vi "WriteFlashFile 3.vi"(0 "Input File Path":path=path "C:/Program Files/WinLapss/Data/4-7-10 2J Anneal Tests/B-615-4-A780_tbilir_Flash-9-5768.dat", 1 "IV array":dbl[][](array[numeric])=[[-0.00396842, -0.00400707, -0.00401566, -0.00399848, -0.00400707, -0.00402855, -0.00398989, -0.00399848, -0.00403713, -0.00402424, -0.00400277, -0.00401137, -0.00396842, -0.00401137, -0.00401566, -0.00395553, -0.00401995, -0.00401995, -0.00400277, -0.00401566, -0.0039856, -0.00401566, -0.00395983, -0.00403284, -0.00400707, -0.00401137, -0.00401137, -0.0039856, -0.00395553, -0.00399419, -0.00403713, -0.00402855, -0.00401995, -0.00397271, -0.0040586, -0.00403713, -0.00396842, -0.00400277, -0.0039813, -0.00404572, -0.0039813, -0.0039856, -0.00403713, -0.00405002, -0.00399848, -0.00399419, -0.00407149, -0.0039813, -0.00402855, -0.00402855, -0.00397701, -0.00399419, -0.00404142, -0.00400707, -0.00399419, -0.00399848, -0.00398989, -0.00400277, -0.00401995, -0.00398989, -0.00402855, -0.00404142, -0.00403713, -0.00404572, -0.00404572, -0.00397271, -0.00399848, -0.00402424, -0.00398989, -0.00403713, -0.00404142, -0.0039813, -0.00402424, -0.00400277, -0.0039813, -0.00402855, -0.00402424, -0.00400277, -0.00404572, -0.00398989, -0.00401137, -0.00400707, -0.00403284, -0.00401995, -0.00408866, -0.00398989, -0.00395553, -0.00395553, -0.00395983, -0.0039856, -0.0039856, -0.00402424, -0.00402855, -0.00401995, -0.00402855, -0.00401995, -0.00402855, -0.00392117, -0.00394266, -0.00399848, -0.00397271, -0.00396413, -0.00403713, -0.00397271, -0.00401137, -0.00404572, -0.00400707, -0.00395553, -0.00401137, -0.00393406, -0.00397701, -0.00405431, -0.0039856, -0.00394266, -0.00402424, -0.00399848, -0.00400707, -0.00403713, -0.00401995, -0.00398989, -0.00400707, -0.00398989, -0.00399848, -0.00397271, -0.00397271, -0.00401137, -0.00402855, -0.00398989, -0.0039813, -0.00399848, -0.00402855, -0.00400707, -0.00407149, -0.00405002, -0.00403284, -0.00401566, -0.00401566, -0.00400277, -0.00401137, -0.00398989, -0.00394695, -0.0039813, -0.00392977, -0.0039856, -0.00398989, -0.00397271, -0.00400277, -0.0039856, -0.00401566, -0.00400707, -0.0039856, -0.00392117, -0.00400277, -0.00398989, -0.00397271, -0.00396413, -0.00397701, -0.00399848, -0.00400277, -0.00395124, -0.00395983, -0.00396413, -0.00396842, -0.00402424, -0.00398989, -0.0039813, -0.00399848, -0.00399848, -0.00394266, -0.00394695, -0.00400707, -0.00401995, -0.00404142, -0.00396413, -0.00400277, -0.00393835, -0.00402855, -0.0039856, -0.0039856, -0.00404572, -0.00400277, -0.00397701, -0.00397701, -0.00396842, -0.00401566, -0.00397271, -0.0039856, -0.00401566, -0.00395124, -0.00400277, -0.00401995, -0.00399419, -0.0039813, -0.00400277, -0.00399848, -0.00396842, -0.00397271, -0.00397271, -0.00396842, -0.00399419, -0.00392117, -0.00392977, -0.0039856, -0.00394266, -0.00395553, -0.00400277, -0.00393406, -0.00396413, -0.00395553, -0.00387824, -0.00393835, -0.00397701, -0.00392548, -0.00395124, -0.00400277, -0.00395983, -0.00400277, -0.00399848, -0.00393406, -0.00395983, -0.0039813, -0.00396413, -0.00394695, -0.00400707, -0.00397271, -0.00397271, -0.00397271, -0.00393406, -0.00394695, -0.00395124, -0.0039856, -0.00397271, -0.00398989, -0.00392548, -0.0039083, -0.00397701, -0.00399419, -0.00389541, -0.0039856, -0.00392977, -0.00396842, -0.00393835, -0.00393406, -0.00395983, -0.00395124, -0.00394266, -0.00397271, -0.00396413, -0.00393406, -0.00395553, -0.00395983, -0.00389112, -0.00392977, -0.00394695, -0.00392117, -0.00395983, -0.00387824, -0.00397701, -0.00395124, -0.00384817, -0.00395124, -0.00396842, -0.00389971, -0.00395124, -0.003904, -0.00386535, -0.00396842, -0.0039083, -0.00385677, -0.00393835, -0.00386964, -0.00392548, -0.00389541, -0.00395124, -0.003904, -0.00396413, -0.00392117, -0.00389541, -0.00391688, -0.00397701, -0.00394695, -0.00394266, -0.00396413, -0.00392977, -0.00397271, -0.00392977, -0.00388253, -0.00392977, -0.00392977, -0.00397701, -0.00392117, -0.00393406, -0.00392117, -0.00395553, -0.00392548, -0.00389971, -0.00392548, -0.00391688, -0.00386106, -0.00388682, -0.00388682, -0.00389112, -0.00392548, -0.00389541, -0.00389971, -0.00391259, -0.0039083, -0.00389541, -0.00384817, -0.00385246, -0.003904, -0.00387394, -0.00386106, -0.00386964, -0.00389541, -0.00387394, -0.00386106, -0.00391259, -0.003904, -0.00382241, -0.00389541, -0.00386106, -0.00385677, -0.00385246, -0.00382241, -0.00387394, -0.00386106, -0.00386106, -0.00385677, -0.00389971, -0.00386106, -0.00385246, -0.00386964, -0.00385677, -0.00387824, -0.00387394, -0.00383528, -0.00387824, -0.00389112, -0.00378805, -0.00383959, -0.00383528, -0.00381382, -0.00379664, -0.00386535, -0.0038267, -0.0038267, -0.0038267, -0.00383528, -0.00388253, -0.00380523, -0.00383528, -0.0038267, -0.00383099, -0.00383528, -0.00377946, -0.00377088, -0.00380523, -0.00377088, -0.00373222, -0.00378805, -0.00380952, -0.00375799, -0.00379235, -0.00376657, -0.00376657, -0.00372792, -0.00373652, -0.00371933, -0.00372363, -0.00372792, -0.00370646, -0.00377517, -0.00371933, -0.00370215, -0.00373222, -0.00368497, -0.00372792, -0.00375799, -0.00368068, -0.00370215, -0.00370646, -0.00369786, -0.0036635, -0.00362486, -0.00368068, -0.00363344, -0.00367639, -0.00361197, -0.00360339, -0.00365492, -0.00359908, -0.00364203, -0.00365062, -0.00357761, -0.00362486, -0.00360339, -0.00359908, -0.00361197, -0.0035905, -0.00356903, -0.00353467, -0.00359908, -0.0035175, -0.00352179, -0.00355614, -0.00347884, -0.00350032, -0.00347884, -0.00341012, -0.00344019, -0.00344448, -0.00339295, -0.00340154, -0.00340583, -0.00338866, -0.00343161, -0.00340583, -0.00331136, -0.00341443, -0.00335001, -0.0032813, -0.00332423, -0.00337577, -0.00328559, -0.00325983, -0.00326841, -0.00322547, -0.00323405, -0.00323834, -0.00320399, -0.00320399, -0.00320399, -0.00315245, -0.0031181, -0.0031224, -0.00307086, -0.0030408, -0.00305798, -0.00302362, -0.0030408, -0.00299785, -0.00289478, -0.00298496, -0.00291625, -0.00290338, -0.00289049, -0.00287331, -0.00285184, -0.00283036, -0.00277025, -0.00274447, -0.00266718, -0.00265858, -0.00266289, -0.00263282, -0.00259846, -0.00258987, -0.00264571, -0.00252975, -0.00251257, -0.00249969, -0.0024138, -0.00238373, -0.00239233, -0.00231931, -0.00231931, -0.00228066, -0.00219477, -0.00219907, -0.00219048, -0.0021003, -0.00208312, -0.00200152, -0.00201441, -0.00193281, -0.00189846, -0.0018598, -0.00182115, -0.00177391, -0.00172237, -0.00167514, -0.00160643, -0.00157207, -0.00149477, -0.00142605, -0.00142176, -0.00130581, -0.00130152, -0.00121562, -0.00119414, -0.00105672, -0.00100089, -0.00101378, -0.000932181, -0.00086776, -0.000790465, -0.000734639, -0.00065304, -0.000580025, -0.00048126, -0.000403953, -0.000365305, -0.000223589, -0.000176346, -0.000111926, 2.11954e-05, 6.84261e-05, 0.000128555, 0.000244498, 0.000360453, 0.000411987, 0.000605226, 0.000609529, 0.000673938, 0.000867188, 0.000901544, 0.0010089, 0.00113773, 0.00124509, 0.00133529, 0.00149847, 0.00163159, 0.00168742, 0.00179908, 0.00191932, 0.00205674, 0.00221564, 0.00236593, 0.002469, 0.00257207, 0.00274385, 0.00284691, 0.00299293, 0.00314323, 0.003242, 0.0033923, 0.00353402, 0.0036972, 0.00393341, 0.00404935, 0.00417389, 0.00434996, 0.00451314, 0.00474933, 0.00484382, 0.00502847, 0.00514443, 0.00536773, 0.00559105, 0.00571128, 0.00589595, 0.00620943, 0.00634686, 0.00652293, 0.00676342, 0.00696526, 0.00709409, 0.0073904, 0.00766095, 0.0077726, 0.00798732, 0.00827935, 0.00841676, 0.00874314, 0.00891062, 0.00916829, 0.00944313, 0.00964067, 0.00986828, 0.0101818, 0.0104566, 0.0106713, 0.0108775, 0.0111566, 0.0114186, 0.0117406, 0.0119811, 0.012286, 0.012548, 0.0128443, 0.0130934, 0.0134584, 0.0137075, 0.0140124, 0.0143774, 0.0146136, 0.0149743, 0.0152535, 0.0156142, 0.0159019, 0.0162412, 0.0165461, 0.0169412, 0.0173277, 0.0175939, 0.0179546, 0.0183454, 0.0187019, 0.0190283, 0.0193718, 0.019754, 0.0200246, 0.0200374, 0.0200117, 0.0200546, 0.0200117, 0.0199816, 0.0199988, 0.0200374, 0.0199902, 0.0199859, 0.0199687, 0.0200246, 0.0199902, 0.0200589, 0.0199902, 0.0199816, 0.020016, 0.0199988, 0.020016, 0.0200203, 0.020016, 0.0200074, 0.0200289, 0.0199902, 0.0200374, 0.0200503, 0.0199988, 0.0200074, 0.0200117, 0.0200503, 0.0199859, 0.019973, 0.0199945, 0.0200117, 0.0200503, 0.0199687, 0.0199902, 0.020016, 0.0200074, 0.0200203, 0.0200074, 0.0200031, 0.0199902, 0.0200117, 0.0199945, 0.0199859, 0.0200031, 0.0199988, 0.0199859, 0.020016, 0.0199945, 0.0199945, 0.0200117, 0.0200074, 0.0199945, 0.020016, 0.019973, 0.0199859, 0.0199902, 0.020016, 0.0199945, 0.0199687, 0.020016, 0.0199902, 0.0199816, 0.0199988, 0.0199902, 0.0199945, 0.0199902, 0.0200203, 0.0200074, 0.0199945, 0.0200417, 0.0199644, 0.0199859, 0.0199988, 0.0199687, 0.0200074, 0.0199859, 0.0200503, 0.0199945, 0.0199988, 0.0200031, 0.0200031, 0.0200289, 0.0200246, 0.0200374, 0.0200589, 0.019973, 0.0200031, 0.0199687, 0.0199945, 0.0199859, 0.0199773, 0.0199902, 0.0199816, 0.0200289, 0.0199859, 0.020016, 0.0199945, 0.0200031, 0.0200203, 0.0199773, 0.0200246, 0.0200246, 0.0200074, 0.0200417, 0.0200203, 0.0200203, 0.0200289, 0.0199988, 0.0199945, 0.0200074, 0.0199601, 0.0199902, 0.0200417, 0.0199773, 0.0199945, 0.0200074, 0.0200031, 0.0199816, 0.0199902, 0.0200031, 0.0200289, 0.0200031, 0.0199988, 0.0199902, 0.0199988, 0.0199945, 0.0200031, 0.0200117, 0.0200031, 0.0199945, 0.0200246, 0.0200031, 0.0200289, 0.0200203, 0.0199945, 0.0199859, 0.0199988, 0.0200117, 0.0200331, 0.0200074, 0.0199988, 0.0199945, 0.0200031, 0.0199988, 0.0199945, 0.0199945, 0.0199988, 0.0199816, 0.0200031, 0.0200031, 0.0199945, 0.019973, 0.0199773, 0.0199988, 0.0200074, 0.019973, 0.0199816, 0.0199773, 0.0200246, 0.019973, 0.0199601, 0.0200031, 0.0199773, 0.0200031, 0.0199988, 0.0200417, 0.0200117, 0.0200203, 0.0200289, 0.0199687, 0.0200417, 0.0200374, 0.0200031, 0.0200117, 0.0199988, 0.0200203, 0.0200031, 0.0199687, 0.0200074, 0.0199859, 0.0199988, 0.020046, 0.0200117, 0.0199902, 0.0200117, 0.0199773, 0.020046, 0.0199816, 0.0199902, 0.0200117, 0.0200289, 0.0200246, 0.0200374, 0.019973, 0.019973, 0.0200289, 0.0199988, 0.0200031, 0.0200031, 0.0199988, 0.0199945, 0.0199687, 0.0200417, 0.0199859, 0.0199773, 0.0200246, 0.0200031, 0.0199816, 0.0199687, 0.0200031, 0.0200031, 0.0200246, 0.0200031, 0.0200289, 0.020016, 0.0199945, 0.0200031, 0.0200117, 0.0199988, 0.0200074, 0.0200289, 0.0199902, 0.0199902, 0.0200503, 0.0199988, 0.0200031, 0.0200031, 0.0199816, 0.0199902, 0.0199988, 0.0200246, 0.0199687, 0.0200246, 0.0199988, 0.0200117, 0.0199988, 0.0199945, 0.020016, 0.0199859, 0.0199945, 0.0200031, 0.0199945, 0.0199988, 0.019973, 0.0199988, 0.0200503, 0.0199644, 0.0199945, 0.020016, 0.0199988, 0.0200031, 0.0199988, 0.0199859, 0.0200503, 0.0200117, 0.0200331, 0.0200374, 0.019973, 0.0199859, 0.0199773, 0.0200031, 0.0200331, 0.0200503, 0.0199988, 0.0200117, 0.0199773, 0.0200031, 0.0199816, 0.0199945, 0.0199902, 0.0200074, 0.0199859, 0.0200117, 0.0200331, 0.0200289, 0.0200031, 0.0199902, 0.0200374, 0.0200074, 0.0199816, 0.019973, 0.0200331, 0.0200031, 0.020016, 0.0200117, 0.0199773, 0.0200117, 0.0200074, 0.0199902, 0.0200246, 0.0199773, 0.020016, 0.0200117, 0.0199859, 0.0199601, 0.0200074, 0.019973, 0.0200074, 0.0200417, 0.0199859, 0.0199773, 0.0200289, 0.0199988, 0.0200331, 0.0199902, 0.0199945, 0.0199773, 0.020016, 0.0199816, 0.0200289, 0.0200246, 0.020016, 0.0200117, 0.0199988, 0.019973, 0.0199902, 0.0199945, 0.0200074, 0.0200117, 0.0200117, 0.0200074, 0.0200417, 0.0199988, 0.0199988, 0.0200117, 0.0199816, 0.0199945, 0.0200074, 0.0199816, 0.0199988, 0.0199859, 0.0199988, 0.0200417, 0.0200074, 0.020016, 0.0200074, 0.0199988, 0.0199859, 0.0199945, 0.0199902, 0.0200074, 0.0199945, 0.0199988, 0.0199945, 0.0199773, 0.0199859, 0.0200117, 0.0200246, 0.0199773, 0.0199988, 0.0199988, 0.0200031, 0.0200074, 0.0199988, 0.0200117, 0.0199902, 0.019973, 0.0199945, 0.0199816, 0.0200031, 0.0200117, 0.0199687, 0.0199816, 0.0200246, 0.020016, 0.0199945, 0.0200117, 0.0200417, 0.0200031, 0.0200074, 0.0199773, 0.020016, 0.020046, 0.0199945, 0.0199902, 0.0200289, 0.0199773, 0.0200246, 0.0200203, 0.0199945, 0.0200203, 0.0199945, 0.0200117, 0.0200417, 0.0200031, 0.0200246, 0.0200331, 0.0200117, 0.0199902, 0.0199945, 0.0200074, 0.0199945, 0.0200031, 0.0199816, 0.0200289, 0.0200074, 0.0199601, 0.0199988, 0.0199816, 0.0200246, 0.0200031, 0.0199687, 0.0200031, 0.0200074, 0.019973, 0.0199859, 0.0200031, 0.0199945, 0.0199945, 0.0199945, 0.0200331, 0.0200031, 0.0199945, 0.0199945, 0.0199988, 0.0199945, 0.0199644, 0.0200117, 0.0199902], [-0.1, -0.09912023460410557, -0.09824046920821115, -0.09736070381231672, -0.09648093841642229, -0.09560117302052787, -0.09472140762463344, -0.093841642228739, -0.09296187683284458, -0.09208211143695015, -0.09120234604105572, -0.0903225806451613, -0.08944281524926687, -0.08856304985337243, -0.08768328445747801, -0.08680351906158358, -0.08592375366568915, -0.08504398826979473, -0.0841642228739003, -0.08328445747800586, -0.08240469208211144, -0.08152492668621701, -0.08064516129032258, -0.07976539589442816, -0.07888563049853373, -0.07800586510263931, -0.07712609970674487, -0.07624633431085044, -0.07536656891495602, -0.07448680351906159, -0.07360703812316716, -0.07272727272727274, -0.0718475073313783, -0.07096774193548387, -0.07008797653958945, -0.06920821114369502, -0.06832844574780059, -0.06744868035190617, -0.06656891495601173, -0.0656891495601173, -0.06480938416422288, -0.06392961876832845, -0.06304985337243402, -0.06217008797653959, -0.061290322580645165, -0.06041055718475074, -0.059530791788856306, -0.05865102639296188, -0.057771260997067454, -0.05689149560117302, -0.056011730205278595, -0.05513196480938417, -0.054252199413489736, -0.05337243401759531, -0.052492668621700884, -0.05161290322580645, -0.050733137829912026, -0.0498533724340176, -0.04897360703812317, -0.04809384164222874, -0.047214076246334315, -0.04633431085043989, -0.045454545454545456, -0.04457478005865103, -0.043695014662756604, -0.04281524926686217, -0.041935483870967745, -0.04105571847507332, -0.040175953079178886, -0.03929618768328446, -0.038416422287390034, -0.0375366568914956, -0.036656891495601175, -0.03577712609970675, -0.034897360703812316, -0.03401759530791789, -0.033137829912023464, -0.03225806451612903, -0.031378299120234605, -0.030498533724340176, -0.02961876832844575, -0.02873900293255132, -0.027859237536656895, -0.026979472140762465, -0.026099706744868036, -0.02521994134897361, -0.02434017595307918, -0.02346041055718475, -0.022580645161290325, -0.021700879765395895, -0.020821114369501466, -0.01994134897360704, -0.01906158357771261, -0.018181818181818184, -0.017302052785923755, -0.016422287390029325, -0.015542521994134898, -0.01466275659824047, -0.013782991202346042, -0.012903225806451613, -0.012023460410557185, -0.011143695014662757, -0.01026392961876833, -0.0093841642228739, -0.008504398826979473, -0.007624633431085044, -0.006744868035190616, -0.005865102639296188, -0.00498533724340176, -0.004105571847507331, -0.0032258064516129032, -0.002346041055718475, -0.001466275659824047, -0.0005865102639296188, 0.0002932551319648094, 0.0011730205278592375, 0.0020527859237536657, 0.002932551319648094, 0.0038123167155425224, 0.00469208211143695, 0.005571847507331379, 0.0064516129032258064, 0.007331378299120235, 0.008211143695014663, 0.009090909090909092, 0.00997067448680352, 0.010850439882697948, 0.011730205278592375, 0.012609970674486805, 0.013489736070381233, 0.01436950146627566, 0.015249266862170088, 0.016129032258064516, 0.017008797653958945, 0.017888563049853375, 0.0187683284457478, 0.01964809384164223, 0.02052785923753666, 0.021407624633431085, 0.022287390029325515, 0.023167155425219944, 0.02404692082111437, 0.0249266862170088, 0.025806451612903226, 0.026686217008797655, 0.027565982404692085, 0.02844574780058651, 0.02932551319648094, 0.03020527859237537, 0.031085043988269796, 0.031964809384164225, 0.03284457478005865, 0.033724340175953084, 0.03460410557184751, 0.035483870967741936, 0.03636363636363637, 0.037243401759530795, 0.03812316715542522, 0.039002932551319654, 0.03988269794721408, 0.040762463343108506, 0.04164222873900293, 0.042521994134897365, 0.04340175953079179, 0.04428152492668622, 0.04516129032258065, 0.046041055718475075, 0.0469208211143695, 0.047800586510263934, 0.04868035190615836, 0.049560117302052786, 0.05043988269794722, 0.051319648093841645, 0.05219941348973607, 0.053079178885630504, 0.05395894428152493, 0.054838709677419356, 0.05571847507331379, 0.056598240469208215, 0.05747800586510264, 0.058357771260997074, 0.0592375366568915, 0.060117302052785926, 0.06099706744868035, 0.061876832844574785, 0.06275659824046921, 0.06363636363636364, 0.06451612903225806, 0.0653958944281525, 0.06627565982404693, 0.06715542521994135, 0.06803519061583578, 0.06891495601173021, 0.06979472140762463, 0.07067448680351907, 0.0715542521994135, 0.07243401759530792, 0.07331378299120235, 0.07419354838709678, 0.0750733137829912, 0.07595307917888564, 0.07683284457478007, 0.07771260997067449, 0.07859237536656892, 0.07947214076246335, 0.08035190615835777, 0.0812316715542522, 0.08211143695014664, 0.08299120234604106, 0.08387096774193549, 0.08475073313782992, 0.08563049853372434, 0.08651026392961877, 0.08739002932551321, 0.08826979472140763, 0.08914956011730206, 0.09002932551319649, 0.09090909090909091, 0.09178885630498534, 0.09266862170087978, 0.0935483870967742, 0.09442815249266863, 0.09530791788856305, 0.09618768328445748, 0.09706744868035191, 0.09794721407624633, 0.09882697947214077, 0.0997067448680352, 0.10058651026392962, 0.10146627565982405, 0.10234604105571848, 0.1032258064516129, 0.10410557184750734, 0.10498533724340177, 0.10586510263929619, 0.10674486803519062, 0.10762463343108505, 0.10850439882697947, 0.1093841642228739, 0.11026392961876834, 0.11114369501466276, 0.11202346041055719, 0.11290322580645162, 0.11378299120234604, 0.11466275659824048, 0.11554252199413491, 0.11642228739002933, 0.11730205278592376, 0.1181818181818182, 0.11906158357771261, 0.11994134897360705, 0.12082111436950148, 0.1217008797653959, 0.12258064516129033, 0.12346041055718476, 0.12434017595307918, 0.1252199413489736, 0.12609970674486803, 0.12697947214076247, 0.1278592375366569, 0.12873900293255133, 0.12961876832844577, 0.13049853372434017, 0.1313782991202346, 0.13225806451612904, 0.13313782991202347, 0.1340175953079179, 0.13489736070381234, 0.13577712609970674, 0.13665689149560117, 0.1375366568914956, 0.13841642228739004, 0.13929618768328447, 0.1401759530791789, 0.1410557184750733, 0.14193548387096774, 0.14281524926686218, 0.1436950146627566, 0.14457478005865104, 0.14545454545454548, 0.14633431085043988, 0.1472140762463343, 0.14809384164222875, 0.14897360703812318, 0.1498533724340176, 0.15073313782991205, 0.15161290322580645, 0.15249266862170088, 0.15337243401759532, 0.15425219941348975, 0.15513196480938418, 0.15601173020527861, 0.15689149560117302, 0.15777126099706745, 0.15865102639296189, 0.15953079178885632, 0.16041055718475075, 0.16129032258064516, 0.1621700879765396, 0.16304985337243402, 0.16392961876832846, 0.1648093841642229, 0.16568914956011732, 0.16656891495601173, 0.16744868035190616, 0.1683284457478006, 0.16920821114369503, 0.17008797653958946, 0.1709677419354839, 0.1718475073313783, 0.17272727272727273, 0.17360703812316716, 0.1744868035190616, 0.17536656891495603, 0.17624633431085046, 0.17712609970674487, 0.1780058651026393, 0.17888563049853373, 0.17976539589442816, 0.1806451612903226, 0.18152492668621703, 0.18240469208211144, 0.18328445747800587, 0.1841642228739003, 0.18504398826979473, 0.18592375366568917, 0.1868035190615836, 0.187683284457478, 0.18856304985337244, 0.18944281524926687, 0.1903225806451613, 0.19120234604105574, 0.19208211143695017, 0.19296187683284458, 0.193841642228739, 0.19472140762463344, 0.19560117302052787, 0.1964809384164223, 0.19736070381231674, 0.19824046920821115, 0.19912023460410558, 0.2, 0.20087976539589444, 0.20175953079178888, 0.20263929618768328, 0.20351906158357772, 0.20439882697947215, 0.20527859237536658, 0.206158357771261, 0.20703812316715545, 0.20791788856304985, 0.20879765395894428, 0.20967741935483872, 0.21055718475073315, 0.21143695014662758, 0.21231671554252202, 0.21319648093841642, 0.21407624633431085, 0.2149560117302053, 0.21583577712609972, 0.21671554252199415, 0.2175953079178886, 0.218475073313783, 0.21935483870967742, 0.22023460410557186, 0.2211143695014663, 0.22199413489736072, 0.22287390029325516, 0.22375366568914956, 0.224633431085044, 0.22551319648093843, 0.22639296187683286, 0.2272727272727273, 0.22815249266862173, 0.22903225806451613, 0.22991202346041056, 0.230791788856305, 0.23167155425219943, 0.23255131964809386, 0.2334310850439883, 0.2343108504398827, 0.23519061583577713, 0.23607038123167157, 0.236950146627566, 0.23782991202346043, 0.23870967741935487, 0.23958944281524927, 0.2404692082111437, 0.24134897360703814, 0.24222873900293257, 0.243108504398827, 0.2439882697947214, 0.24486803519061584, 0.24574780058651027, 0.2466275659824047, 0.24750733137829914, 0.24838709677419357, 0.24926686217008798, 0.25014662756598244, 0.25102639296187684, 0.25190615835777125, 0.2527859237536657, 0.2536656891495601, 0.2545454545454546, 0.255425219941349, 0.25630498533724344, 0.25718475073313785, 0.25806451612903225, 0.2589442815249267, 0.2598240469208211, 0.2607038123167156, 0.26158357771261, 0.2624633431085044, 0.26334310850439885, 0.26422287390029325, 0.2651026392961877, 0.2659824046920821, 0.2668621700879766, 0.267741935483871, 0.2686217008797654, 0.26950146627565985, 0.27038123167155426, 0.2712609970674487, 0.2721407624633431, 0.2730205278592375, 0.273900293255132, 0.2747800586510264, 0.27565982404692085, 0.27653958944281526, 0.2774193548387097, 0.2782991202346041, 0.27917888563049853, 0.280058651026393, 0.2809384164222874, 0.28181818181818186, 0.28269794721407626, 0.28357771260997067, 0.2844574780058651, 0.28533724340175953, 0.286217008797654, 0.2870967741935484, 0.2879765395894428, 0.28885630498533726, 0.28973607038123167, 0.29061583577712613, 0.29149560117302054, 0.292375366568915, 0.2932551319648094, 0.2941348973607038, 0.29501466275659827, 0.2958944281524927, 0.29677419354838713, 0.29765395894428154, 0.29853372434017594, 0.2994134897360704, 0.3002932551319648, 0.30117302052785927, 0.3020527859237537, 0.30293255131964814, 0.30381231671554254, 0.30469208211143695, 0.3055718475073314, 0.3064516129032258, 0.3073313782991203, 0.3082111436950147, 0.3090909090909091, 0.30997067448680354, 0.31085043988269795, 0.3117302052785924, 0.3126099706744868, 0.3134897360703813, 0.3143695014662757, 0.3152492668621701, 0.31612903225806455, 0.31700879765395895, 0.3178885630498534, 0.3187683284457478, 0.3196480938416422, 0.3205278592375367, 0.3214076246334311, 0.32228739002932555, 0.32316715542521995, 0.3240469208211144, 0.3249266862170088, 0.3258064516129032, 0.3266862170087977, 0.3275659824046921, 0.32844574780058655, 0.32932551319648096, 0.33020527859237536, 0.3310850439882698, 0.33196480938416423, 0.3328445747800587, 0.3337243401759531, 0.3346041055718475, 0.33548387096774196, 0.33636363636363636, 0.3372434017595308, 0.33812316715542523, 0.3390029325513197, 0.3398826979472141, 0.3407624633431085, 0.34164222873900296, 0.34252199413489737, 0.34340175953079183, 0.34428152492668623, 0.34516129032258064, 0.3460410557184751, 0.3469208211143695, 0.34780058651026396, 0.34868035190615837, 0.34956011730205283, 0.35043988269794724, 0.35131964809384164, 0.3521994134897361, 0.3530791788856305, 0.35395894428152497, 0.3548387096774194, 0.3557184750733138, 0.35659824046920824, 0.35747800586510264, 0.3583577712609971, 0.3592375366568915, 0.36011730205278597, 0.3609970674486804, 0.3618768328445748, 0.36275659824046924, 0.36363636363636365, 0.3645161290322581, 0.3653958944281525, 0.3662756598240469, 0.3671554252199414, 0.3680351906158358, 0.36891495601173024, 0.36979472140762465, 0.3706744868035191, 0.3715542521994135, 0.3724340175953079, 0.3733137829912024, 0.3741935483870968, 0.37507331378299125, 0.37595307917888565, 0.37683284457478006, 0.3777126099706745, 0.3785923753665689, 0.3794721407624634, 0.3803519061583578, 0.3812316715542522, 0.38211143695014665, 0.38299120234604106, 0.3838709677419355, 0.3847507331378299, 0.3856304985337244, 0.3865102639296188, 0.3873900293255132, 0.38826979472140766, 0.38914956011730206, 0.3900293255131965, 0.39090909090909093, 0.39178885630498533, 0.3926686217008798, 0.3935483870967742, 0.39442815249266866, 0.39530791788856307, 0.3961876832844575, 0.39706744868035193, 0.39794721407624634, 0.3988269794721408, 0.3997067448680352, 0.40058651026392966, 0.40146627565982407, 0.4023460410557185, 0.40322580645161293, 0.40410557184750734, 0.4049853372434018, 0.4058651026392962, 0.40674486803519067, 0.40762463343108507, 0.4085043988269795, 0.40938416422287394, 0.41026392961876834, 0.4111436950146628, 0.4120234604105572, 0.4129032258064516, 0.4137829912023461, 0.4146627565982405, 0.41554252199413494, 0.41642228739002934, 0.41730205278592375, 0.4181818181818182, 0.4190615835777126, 0.4199413489736071, 0.4208211143695015, 0.42170087976539594, 0.42258064516129035, 0.42346041055718475, 0.4243401759530792, 0.4252199413489736, 0.4260997067448681, 0.4269794721407625, 0.4278592375366569, 0.42873900293255135, 0.42961876832844575, 0.4304985337243402, 0.4313782991202346, 0.4322580645161291, 0.4331378299120235, 0.4340175953079179, 0.43489736070381235, 0.43577712609970676, 0.4366568914956012, 0.4375366568914956, 0.43841642228739003, 0.4392961876832845, 0.4401759530791789, 0.44105571847507336, 0.44193548387096776, 0.4428152492668622, 0.4436950146627566, 0.44457478005865103, 0.4454545454545455, 0.4463343108504399, 0.44721407624633436, 0.44809384164222876, 0.44897360703812317, 0.44985337243401763, 0.45073313782991203, 0.4516129032258065, 0.4524926686217009, 0.45337243401759536, 0.45425219941348977, 0.45513196480938417, 0.45601173020527863, 0.45689149560117304, 0.4577712609970675, 0.4586510263929619, 0.4595307917888563, 0.46041055718475077, 0.4612903225806452, 0.46217008797653963, 0.46304985337243404, 0.46392961876832844, 0.4648093841642229, 0.4656891495601173, 0.46656891495601177, 0.4674486803519062, 0.46832844574780064, 0.46920821114369504, 0.47008797653958945, 0.4709677419354839, 0.4718475073313783, 0.4727272727272728, 0.4736070381231672, 0.4744868035190616, 0.47536656891495604, 0.47624633431085045, 0.4771260997067449, 0.4780058651026393, 0.4788856304985338, 0.4797653958944282, 0.4806451612903226, 0.48152492668621705, 0.48240469208211145, 0.4832844574780059, 0.4841642228739003, 0.4850439882697947, 0.4859237536656892, 0.4868035190615836, 0.48768328445747805, 0.48856304985337246, 0.4894428152492669, 0.4903225806451613, 0.4912023460410557, 0.4920821114369502, 0.4929618768328446, 0.49384164222873905, 0.49472140762463346, 0.49560117302052786, 0.4964809384164223, 0.49736070381231673, 0.4982404692082112, 0.4991202346041056, 0.5, 0.5008797653958944, 0.5017595307917889, 0.5026392961876833, 0.5035190615835777, 0.5043988269794721, 0.5052785923753665, 0.5061583577712611, 0.5070381231671555, 0.5079178885630499, 0.5087976539589443, 0.5096774193548388, 0.5105571847507332, 0.5114369501466276, 0.512316715542522, 0.5131964809384164, 0.5140762463343109, 0.5149560117302053, 0.5158357771260997, 0.5167155425219941, 0.5175953079178885, 0.5184750733137831, 0.5193548387096775, 0.5202346041055719, 0.5211143695014663, 0.5219941348973607, 0.5228739002932552, 0.5237536656891496, 0.524633431085044, 0.5255131964809384, 0.5263929618768328, 0.5272727272727273, 0.5281524926686217, 0.5290322580645161, 0.5299120234604106, 0.5307917888563051, 0.5316715542521995, 0.5325513196480939, 0.5334310850439883, 0.5343108504398827, 0.5351906158357772, 0.5360703812316716, 0.536950146627566, 0.5378299120234604, 0.5387096774193548, 0.5395894428152493, 0.5404692082111437, 0.5413489736070382, 0.5422287390029326, 0.543108504398827, 0.5439882697947215, 0.5448680351906159, 0.5457478005865103, 0.5466275659824047, 0.5475073313782991, 0.5483870967741936, 0.549266862170088, 0.5501466275659824, 0.5510263929618768, 0.5519061583577712, 0.5527859237536658, 0.5536656891495602, 0.5545454545454546, 0.555425219941349, 0.5563049853372435, 0.5571847507331379, 0.5580645161290323, 0.5589442815249267, 0.5598240469208211, 0.5607038123167156, 0.56158357771261, 0.5624633431085044, 0.5633431085043988, 0.5642228739002932, 0.5651026392961878, 0.5659824046920822, 0.5668621700879766, 0.567741935483871, 0.5686217008797654, 0.5695014662756599, 0.5703812316715543, 0.5712609970674487, 0.5721407624633431, 0.5730205278592375, 0.573900293255132, 0.5747800586510264, 0.5756598240469208, 0.5765395894428152, 0.5774193548387098, 0.5782991202346042, 0.5791788856304986, 0.580058651026393, 0.5809384164222874, 0.5818181818181819, 0.5826979472140763, 0.5835777126099707, 0.5844574780058651, 0.5853372434017595, 0.586217008797654, 0.5870967741935484, 0.5879765395894428, 0.5888563049853373, 0.5897360703812317, 0.5906158357771262, 0.5914956011730206, 0.592375366568915, 0.5932551319648094, 0.5941348973607038, 0.5950146627565983, 0.5958944281524927, 0.5967741935483871, 0.5976539589442815, 0.5985337243401759, 0.5994134897360704, 0.6002932551319649, 0.6011730205278593, 0.6020527859237537, 0.6029325513196482, 0.6038123167155426, 0.604692082111437, 0.6055718475073314, 0.6064516129032258, 0.6073313782991203, 0.6082111436950147, 0.6090909090909091, 0.6099706744868035, 0.6108504398826979, 0.6117302052785925, 0.6126099706744869, 0.6134897360703813, 0.6143695014662757, 0.6152492668621701, 0.6161290322580646, 0.617008797653959, 0.6178885630498534, 0.6187683284457478, 0.6196480938416422, 0.6205278592375367, 0.6214076246334311, 0.6222873900293255, 0.6231671554252199, 0.6240469208211145, 0.6249266862170089, 0.6258064516129033, 0.6266862170087977, 0.6275659824046921, 0.6284457478005866, 0.629325513196481, 0.6302052785923754, 0.6310850439882698, 0.6319648093841642, 0.6328445747800587, 0.6337243401759531, 0.6346041055718475, 0.635483870967742, 0.6363636363636364, 0.6372434017595309, 0.6381231671554253, 0.6390029325513197, 0.6398826979472141, 0.6407624633431085, 0.641642228739003, 0.6425219941348974, 0.6434017595307918, 0.6442815249266862, 0.6451612903225806, 0.6460410557184751, 0.6469208211143695, 0.647800586510264, 0.6486803519061584, 0.6495601173020529, 0.6504398826979473, 0.6513196480938417, 0.6521994134897361, 0.6530791788856305, 0.653958944281525, 0.6548387096774194, 0.6557184750733138, 0.6565982404692082, 0.6574780058651026, 0.6583577712609971, 0.6592375366568916, 0.660117302052786, 0.6609970674486804, 0.6618768328445748, 0.6627565982404693, 0.6636363636363637, 0.6645161290322581, 0.6653958944281525, 0.6662756598240469, 0.6671554252199414, 0.6680351906158358, 0.6689149560117302, 0.6697947214076246, 0.6706744868035192, 0.6715542521994136, 0.672434017595308, 0.6733137829912024, 0.6741935483870968, 0.6750733137829913, 0.6759530791788857, 0.6768328445747801, 0.6777126099706745, 0.6785923753665689, 0.6794721407624634, 0.6803519061583578, 0.6812316715542522, 0.6821114369501466, 0.682991202346041, 0.6838709677419356, 0.68475073313783, 0.6856304985337244, 0.6865102639296188, 0.6873900293255132, 0.6882697947214077, 0.6891495601173021, 0.6900293255131965, 0.6909090909090909, 0.6917888563049853, 0.6926686217008798, 0.6935483870967742, 0.6944281524926686, 0.695307917888563, 0.6961876832844576, 0.697067448680352, 0.6979472140762464, 0.6988269794721408, 0.6997067448680352, 0.7005865102639297, 0.7014662756598241, 0.7023460410557185, 0.7032258064516129, 0.7041055718475073, 0.7049853372434018, 0.7058651026392962, 0.7067448680351907, 0.7076246334310851, 0.7085043988269795, 0.709384164222874, 0.7102639296187684, 0.7111436950146628, 0.7120234604105572, 0.7129032258064516, 0.7137829912023461, 0.7146627565982405, 0.7155425219941349, 0.7164222873900293, 0.7173020527859237, 0.7181818181818183, 0.7190615835777127, 0.7199413489736071, 0.7208211143695015, 0.721700879765396, 0.7225806451612904, 0.7234604105571848, 0.7243401759530792, 0.7252199413489736, 0.7260997067448681, 0.7269794721407625, 0.7278592375366569, 0.7287390029325513, 0.7296187683284457, 0.7304985337243403, 0.7313782991202347, 0.7322580645161291, 0.7331378299120235, 0.7340175953079179, 0.7348973607038124, 0.7357771260997068, 0.7366568914956012, 0.7375366568914956, 0.73841642228739, 0.7392961876832845, 0.7401759530791789, 0.7410557184750733, 0.7419354838709677, 0.7428152492668623, 0.7436950146627567, 0.7445747800586511, 0.7454545454545455, 0.7463343108504399, 0.7472140762463344, 0.7480938416422288, 0.7489736070381232, 0.7498533724340176, 0.750733137829912, 0.7516129032258065, 0.7524926686217009, 0.7533724340175953, 0.7542521994134898, 0.7551319648093842, 0.7560117302052787, 0.7568914956011731, 0.7577712609970675, 0.7586510263929619, 0.7595307917888563, 0.7604105571847508, 0.7612903225806452, 0.7621700879765396, 0.763049853372434, 0.7639296187683284, 0.764809384164223, 0.7656891495601174, 0.7665689149560118, 0.7674486803519062, 0.7683284457478007, 0.7692082111436951, 0.7700879765395895, 0.7709677419354839, 0.7718475073313783, 0.7727272727272728, 0.7736070381231672, 0.7744868035190616, 0.775366568914956, 0.7762463343108504, 0.777126099706745, 0.7780058651026394, 0.7788856304985338, 0.7797653958944282, 0.7806451612903226, 0.7815249266862171, 0.7824046920821115, 0.7832844574780059, 0.7841642228739003, 0.7850439882697947, 0.7859237536656892, 0.7868035190615836, 0.787683284457478, 0.7885630498533724, 0.789442815249267, 0.7903225806451614, 0.7912023460410558, 0.7920821114369502, 0.7929618768328446, 0.7938416422287391, 0.7947214076246335, 0.7956011730205279, 0.7964809384164223, 0.7973607038123167, 0.7982404692082112, 0.7991202346041056, 0.8]], 2 "Cell Designation":string="SL002", 3 "Current Session":timestamp=timestamp(3388091786.578125 s since 1904-01-01), 4 "Parameters":T8 {"Voc" format="%#_4g"; "Isc" format="%#_4g"; "FF" format="%#_4g"; "Imax" format="%#_4g"; "Vmax" format="%#_4g"; "Pmax" format="%#_4g"; "Itest" format="%#_4g"}, 5 "Light Correction":string="J2", 6 "User":string(combo)="tsun", 7 "Coords":cluster{"Xcoord":dbl, "Ycoord":dbl}={"Xcoord"=3344.0, "Ycoord"=10162.0}, 8 "Package designation":T2, 9 "Bad Flash Info":T1, 10 "Wafer":string="C-160-4-A780", 11 "Wafer Info":T6={"Cell Name (Automatic)"="5500_99_03p5", "Package"="", "Coating"="FOR_AIR", "Comment"="J1 Iso Dual Flash 1697/61", "Flash Setup"="5500_99_03p5", "Hrs under test"=0.0}, 12 "Mask Name":string(combo)="SL002", 13 "CalcValues":T7={"GivenRatio"=0.9694525769209522, "MeasuredRatio"=0.980582402160318, "TopSuns"=595.4283117793674, "MiddleSuns"=588.6700699038504, "ErrorTop"=-0.040824369064393774, "ErrorMiddle"=-0.9200528439605747, "Error Bottom"=0.22541188070332374, "BottomSuns"=100.00691938458719} {"Error Bottom" format="%.2g"; "ErrorMiddle" format="%.2f"; "ErrorTop" format="%.2f"; "MiddleSuns" format="%#.3f"; "TopSuns" format="%#.3f"; "MeasuredRatio" format="%#.3f"; "GivenRatio" format="%#.3f"}, 14 "Temp Data":T5={"Ambient Temperature"=25.91373127207957, "Chuck Set Temperature"=25.91373127207957} {"Chuck Set Temperature" format="%#.1g"; "Ambient Temperature" format="%#.1g"}, 15 "Die Number":string, 16 "Current Device":i32=1, 17 "Data Outputs":T4={"Voc Fit"=3.3458399116005184, "Voc Reg"=3.3461825416563045, "Rs (Ohms)"=0.0, "Rsh"=0.0} {"Rsh" format="%#.6g"; "Voc Fit" format="%0.4f"}, 18 "ConcentrationValues":T3={"Concentration:"=1.0, "Top Current:"=0.00725, "Middle Current:"=0.00488, "Bottom Current:"=0.00826} caption="Calibration values" {"Bottom Current:" format="%#_6p"; "Middle Current:" format="%#_6p"; "Top Current:" format="%#_6p"; "Concentration:" format="%#_6p"}) -> (19 "error out":errorcluster)   [LabVIEW 2012]
panel:
  out "x":string
  out "y":string
  in  "error in":errorcluster caption="error out"
  out "Date/Time string":string="Date: 4/2/2009 12:01 PM"
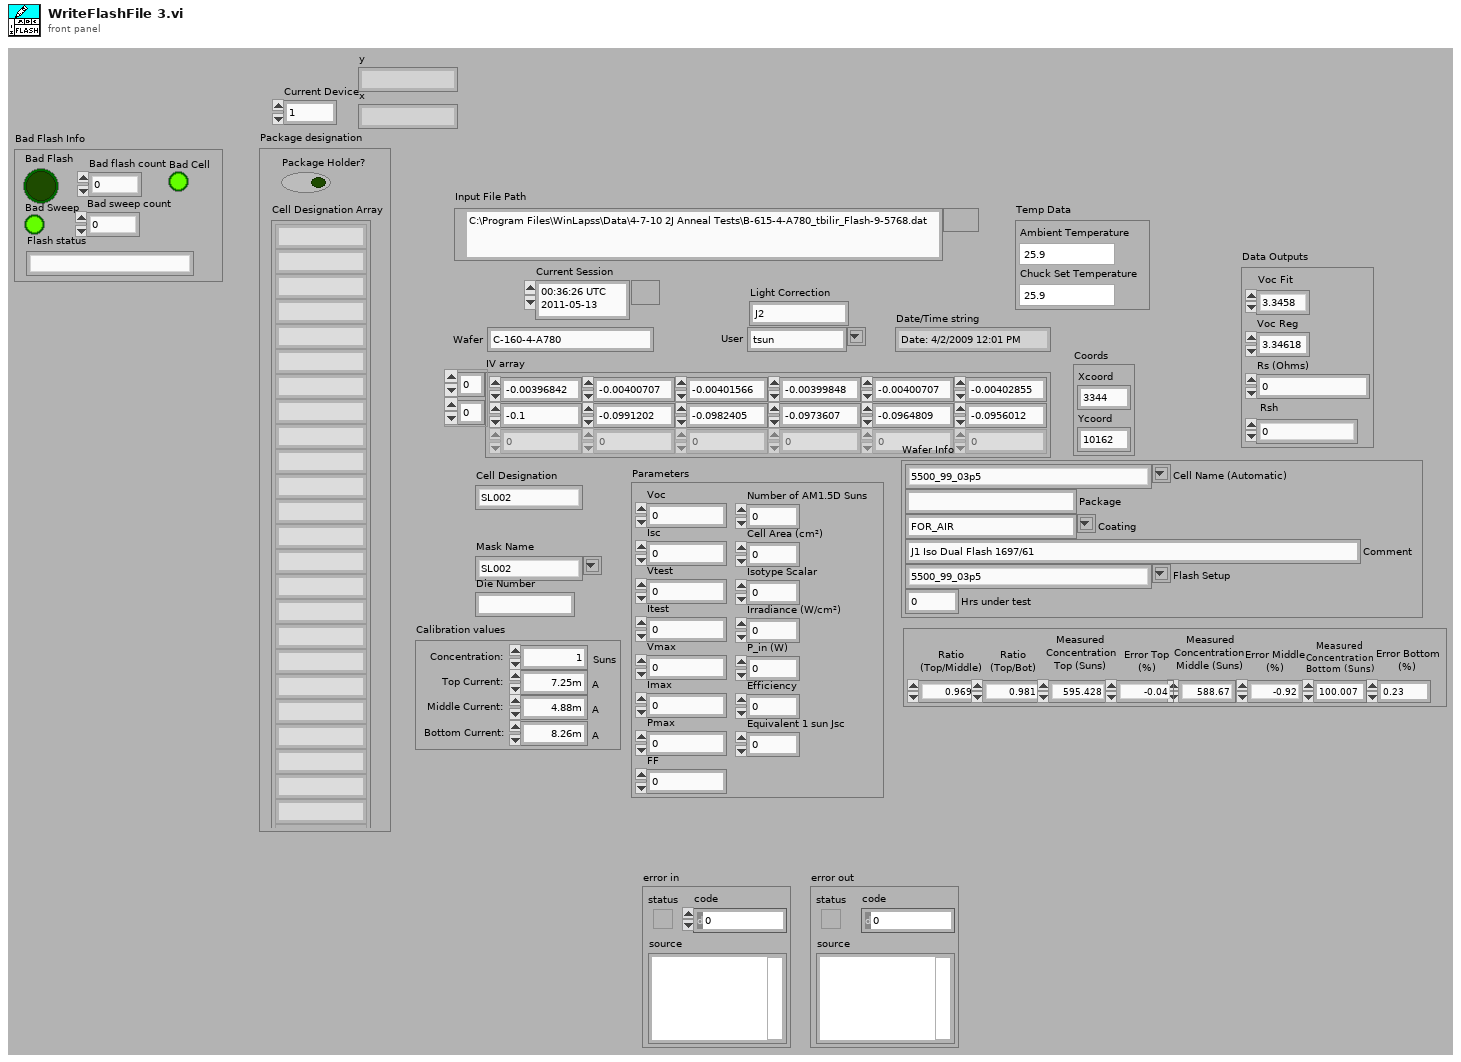
[diagram p1: front panel]
types:
  T1 = cluster{"Bad Flash":bool, "Flash status":string, "Bad Sweep":bool, "Bad flash count":i32, "Bad sweep count":i32, "Bad Cell":bool}
  T2 = cluster{"Package Holder?":bool, "Cell Designation Array":string[]}
  T3 = cluster{"Concentration:":dbl, "Top Current:":dbl, "Middle Current:":dbl, "Bottom Current:":dbl}
  T4 = cluster{"Voc Fit":dbl, "Voc Reg":dbl, "Rs (Ohms)":dbl, "Rsh":dbl}
  T5 = cluster{"Ambient Temperature":dbl, "Chuck Set Temperature":dbl}
  T6 = cluster{"Cell Name (Automatic)":string, "Package":string, "Coating":string, "Comment":string, "Flash Setup":string, "Hrs under test":dbl}
  T7 = cluster{"GivenRatio":dbl, "MeasuredRatio":dbl, "TopSuns":dbl, "MiddleSuns":dbl, "ErrorTop":dbl, "ErrorMiddle":dbl, "Error Bottom":dbl, "BottomSuns":dbl}
  T8 = cluster{"Voc":dbl, "Isc":dbl, "FF":dbl, "Vtest":dbl, "Imax":dbl, "Vmax":dbl, "Pmax":dbl, "Itest":dbl, "Efficiency":dbl, "P_in (W)":dbl, "Irradiance (W/cm²)":dbl, "Cell Area (cm²)":dbl, "Number of AM1.5D Suns":dbl, "Isotype Scalar":dbl, "Equivalent 1 sun Jsc":dbl}
  T9 = enum16{"open", "replace", "create", "open or create", "replace or create", "replace or create with confirmation"}
  T10 = cluster{"3J Ref Current:":dbl, "J1/Top Current:":dbl, "J2/Middle Current:":dbl, "J3/Bottom Current:":dbl, "3J Ref 2 Current:":dbl}
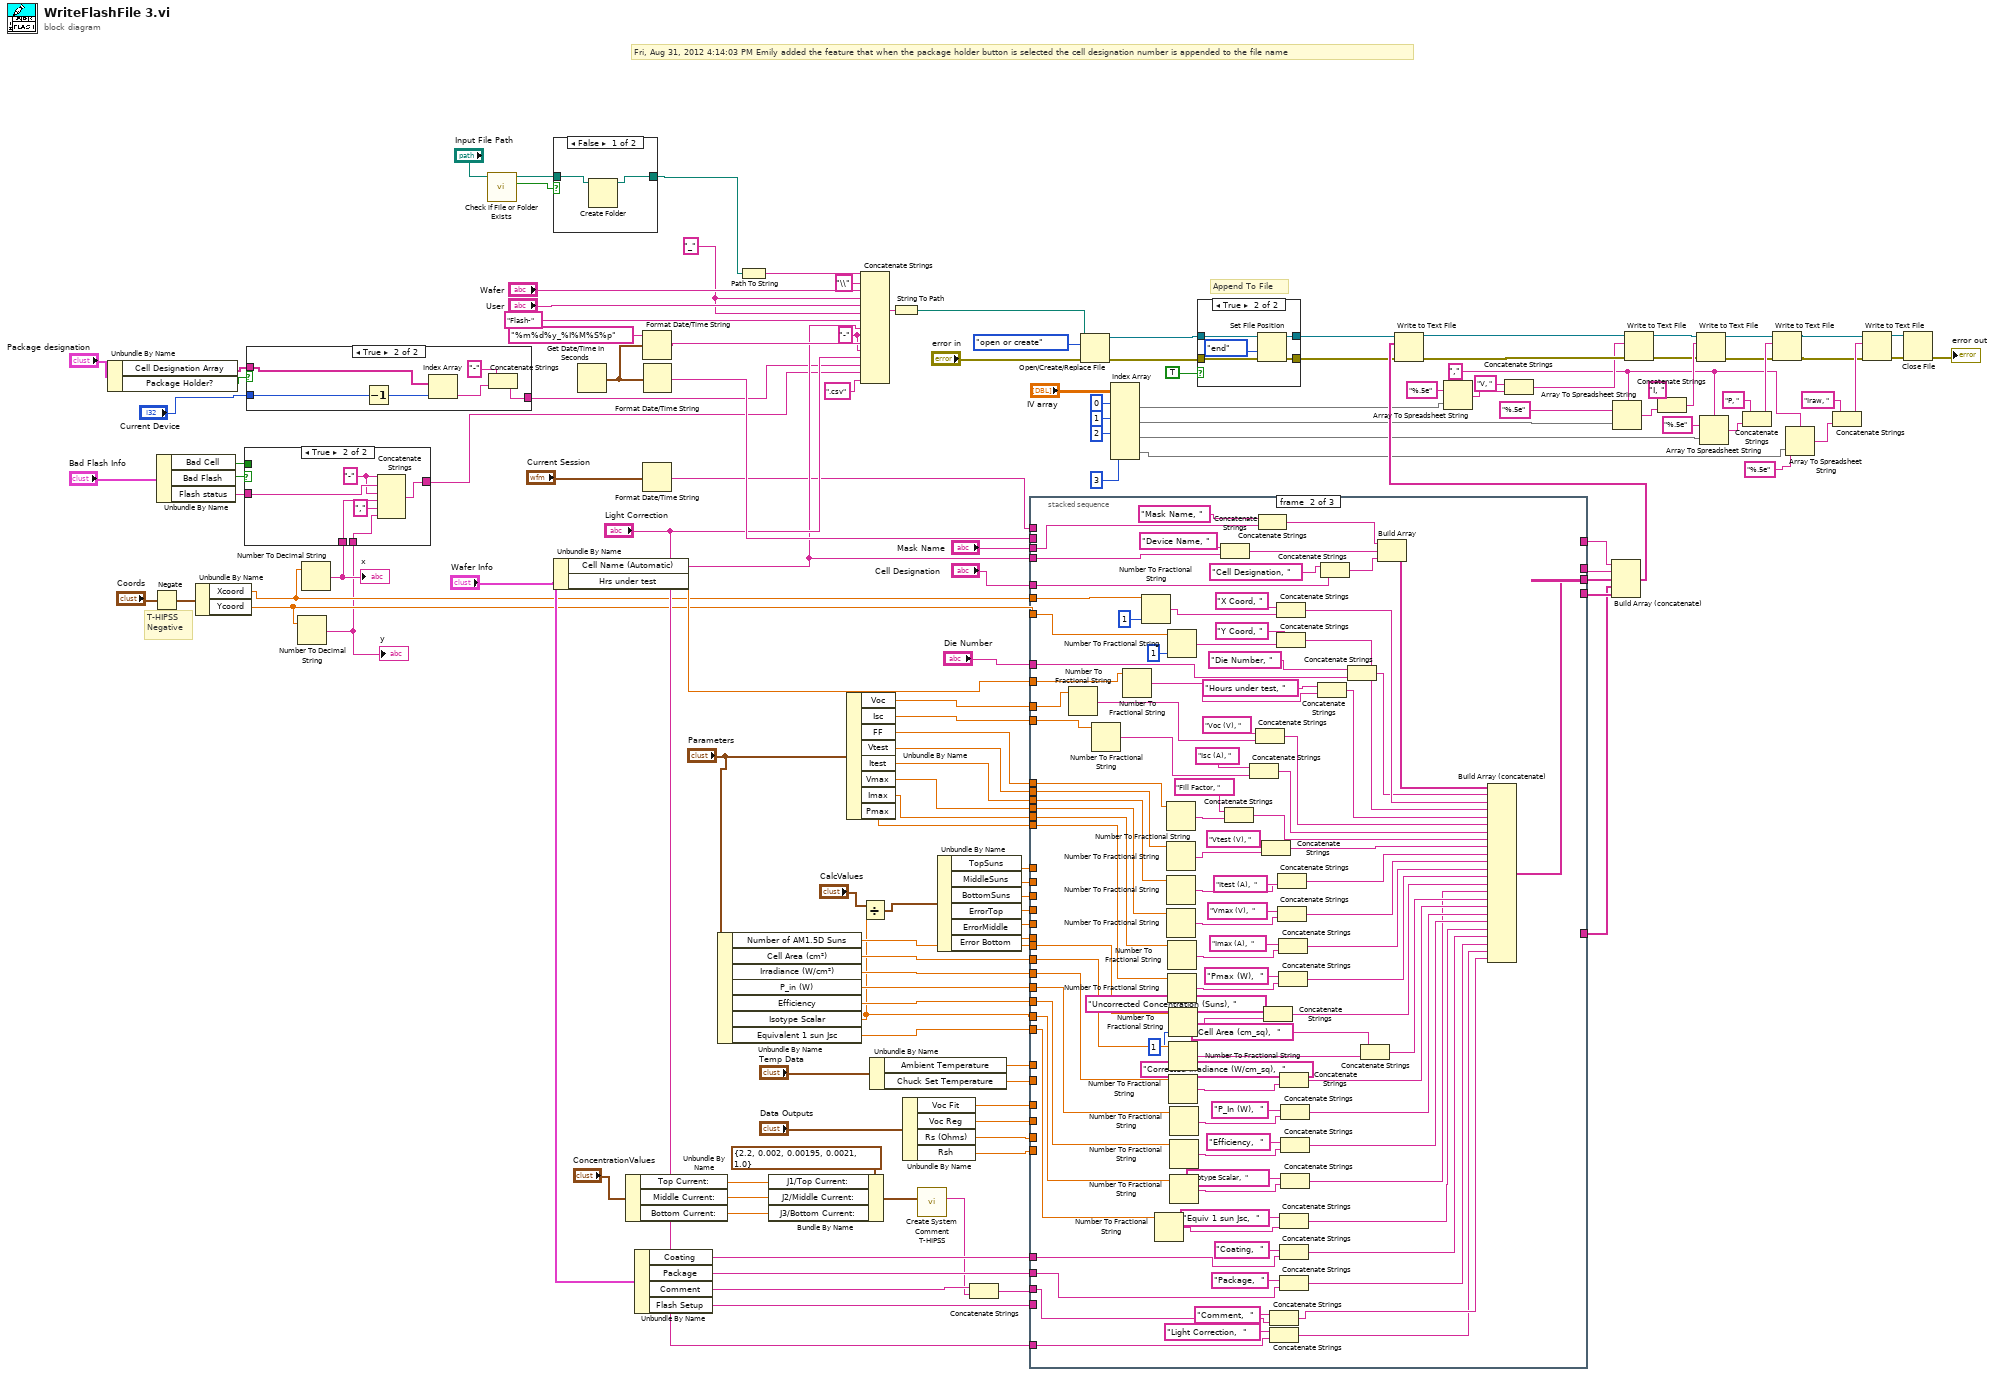
[diagram p0: block diagram]
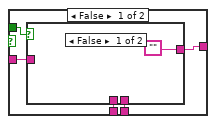
[diagram p3: hidden frame]
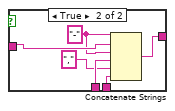
[diagram p4: hidden frame]
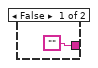
[diagram p5: hidden frame]
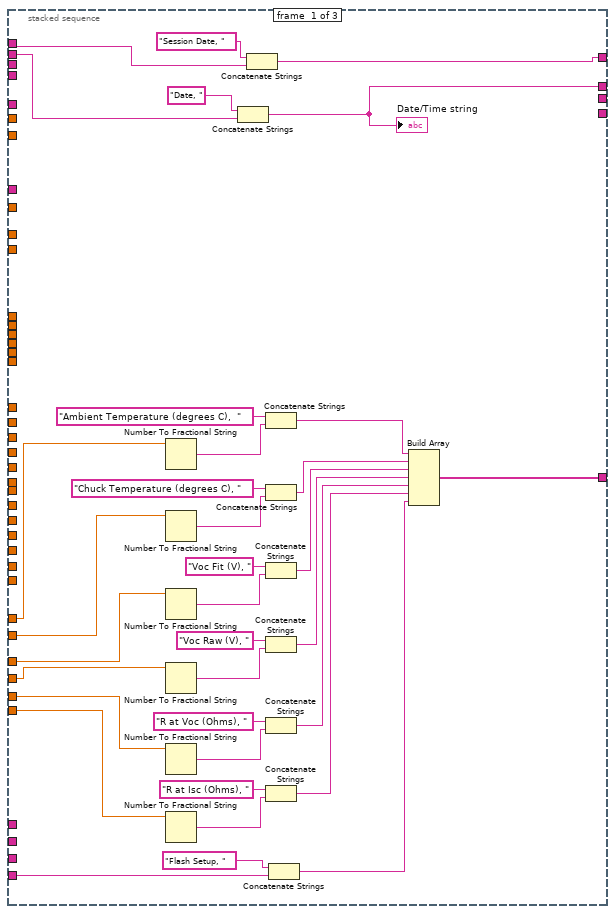
[diagram p7: hidden frame]
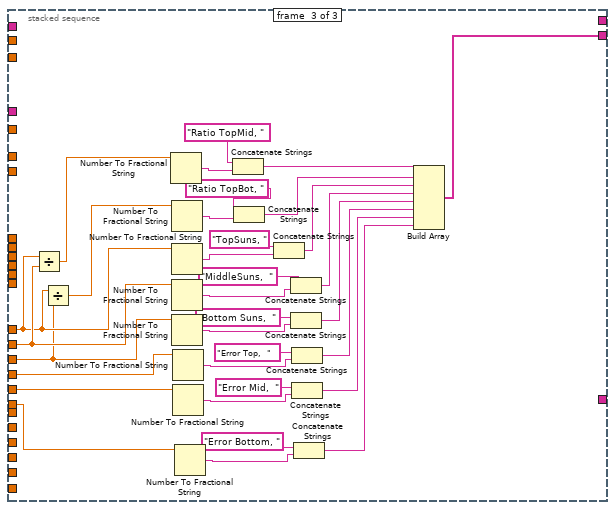
[diagram p8: hidden frame]
diagram:
  w2 = "," ("delimiter (Tab)")
  w56 = "-" ("string")
  w101 = "_" ("string")
  # "Append To File"
  # "Fri, Aug 31, 2012 4:14:03 PM Emily added the feature that when the package holder button is selected the cell designation number is appended to the file name"
  # "T-HIPSS\nNegative"
  n1 = Unbundle By Name("Package designation") -> ("Cell Designation Array"=w50:string[], "Package Holder?"=w51:bool)
  n2 = Negate(x="Coords") -> (-x=w69:cluster{"Xcoord":dbl, "Ycoord":dbl})
  n3 = Unbundle By Name("Bad Flash Info") -> ("Bad Cell"=w47:bool, "Bad Flash"=w54:bool, "Flash status"=w53:string)
  n4 = Unbundle By Name(w69) -> ("Xcoord"=w46:dbl, "Ycoord"=w44:dbl)
  n5 = case shown="True" w51 {
    tunnel: ["" w144] -> w57
    tunnel: "Current Device" -> [_ w140]
    tunnel: w50 -> [_ w139]
    frame False {
    }
    frame True {
      n6 = Decrement(x=w140) -> (x-1=w141:i32)
      n7 = Index Array(array=w139, index=w141) -> (element=w143:string)
      n8 = Concatenate Strings("-", w143) -> (w144:string)
    }
  }
  n9 = Number To Decimal String(number=w44) -> (decimal integer string=w43:string)  [unwired: 1 in]
  "y" <- w43
  n10 = Number To Decimal String(number=w46) -> (decimal integer string=w45:string)  [unwired: 1 in]
  "x" <- w45
  n11 = case shown="True" w54 {
    tunnel: [w147 w162] -> w55
    tunnel: w53 -> [w148 w161]
    tunnel: w47 -> [w149 _]
    tunnel: w45 -> [w146 w159]
    tunnel: w43 -> [w145 w157]
    frame False {
      n12 = case shown="False" w149 {
        tunnel: w148 -> [_ w156]
        tunnel: ["" w151] -> w147
        tunnel: w146 -> [_ w154]
        tunnel: w145 -> [_ w152]
        frame False {
        }
        frame True {
          w155 = "-"
          n13 = Concatenate Strings(w155, w156, w155, w154, ",", w152) -> (w151:string)
        }
      }
    }
    frame True {
      w160 = "-"
      n14 = Concatenate Strings(w160, w161, w160, w159, "," ("string"), w157) -> (w162:string)
    }
  }
  n15 = call <vilib>:"Check if File or Folder Exists.vi"("path"="Input File Path") -> ("file or folder exists?"=w90:bool, "dup path"=w91:path)  [unwired: 1 in, 8 out]
  n16 = case shown="False" w90 {
    tunnel: [w163 w165] -> w92
    tunnel: w91 -> [w164 w165]
    frame False {
      n17 = Create Folder(path (use dialog)=w164) -> (created path=w163:path)  [unwired: 1 in, 3 out]
    }
    frame True {
    }
  }
  n18 = Unbundle By Name("Wafer Info") -> ("Cell Name (Automatic)"=w85:string, "Hrs under test"=w58:dbl)
  n19 = Get Date/Time In Seconds() -> (seconds since 1Jan1904=w95:timestamp)
  n20 = Unbundle By Name("ConcentrationValues") -> ("Top Current:"=w63:dbl, "Middle Current:"=w62:dbl, "Bottom Current:"=w61:dbl)
  n21 = Unbundle By Name("Wafer Info") -> ("Coating"=w120:string, "Package"=w119:string, "Comment"=w67:string, "Flash Setup"=w83:string)
  n22 = Format Date/Time String(time format string (%c)="%m%d%y_%I%M%S%p", seconds (now)=w95) -> (date/time string=w93:string)  [unwired: 1 out]
  n23 = Format Date/Time String(seconds (now)="Current Session") -> (date/time string=w72:string)  [unwired: 2 out]
  n24 = Format Date/Time String(seconds (now)=w95) -> (date/time string=w87:string)  [unwired: 2 out]
  n25 = Unbundle By Name("Parameters") -> ("Number of AM1.5D Suns"=w126:dbl, "Cell Area (cm²)"=w125:dbl, "Irradiance (W/cm²)"=w124:dbl, "P_in (W)"=w123:dbl, "Efficiency"=w122:dbl, "Isotype Scalar"=w110:dbl, "Equivalent 1 sun Jsc"=w121:dbl)
  n26 = Path To String(path=w92) -> (string=w100:string)
  n27 = Bundle By Name(cluster=T10 {"3J Ref Current:"=2.2, "J1/Top Current:"=0.002, "J2/Middle Current:"=0.00195, "J3/Bottom Current:"=0.0021, "3J Ref 2 Current:"=1.0} ("Calibration Values"), "J1/Top Current:"=w63, "J2/Middle Current:"=w62, "J3/Bottom Current:"=w61) -> (w60:T10)
  n28 = Unbundle By Name("Parameters") -> ("Voc"=w136:dbl, "Isc"=w135:dbl, "FF"=w132:dbl, "Vtest"=w131:dbl, "Itest"=w130:dbl, "Vmax"=w129:dbl, "Imax"=w128:dbl, "Pmax"=w127:dbl)
  n29 = Concatenate Strings(w100, "\\" ("string"), "Wafer", w101, "User", w101, "Flash-", w85, w56, w93, w56, "Light Correction", w57, w55, ".csv" ("string")) -> (w98:string)
  n30 = Divide(x="CalcValues", y=w110) -> (x/y=w104:T7)
  n31 = Unbundle By Name("Temp Data") -> ("Ambient Temperature"=w79:dbl, "Chuck Set Temperature"=w78:dbl)
  n32 = String To Path(string=w98) -> (path=w88:path)
  n33 = Unbundle By Name("Data Outputs") -> ("Voc Fit"=w77:dbl, "Voc Reg"=w76:dbl, "Rs (Ohms)"=w75:dbl, "Rsh"=w74:dbl)
  n34 = call "Create System Comment T-HIPSS.vi"("Calibration Values"=w60) -> ("System Comment"=w66:string)  [unwired: 10 in]
  n35 = Unbundle By Name(w104) -> ("TopSuns"=w116:dbl, "MiddleSuns"=w115:dbl, "BottomSuns"=w114:dbl, "ErrorTop"=w113:dbl, "ErrorMiddle"=w112:dbl, "Error Bottom"=w111:dbl)
  n36 = Concatenate Strings(w67, w66) -> (w68:string)
  n37 = stacked-sequence {
    tunnel: [_ w300 _] -> w134
    tunnel: w44 -> [_ w298 _]
    tunnel: w46 -> [_ w299 _]
    tunnel: w136 -> [_ w277 _]
    tunnel: w135 -> [_ w276 _]
    tunnel: "Mask Name" -> [_ w282 _]
    tunnel: [w199 _ _] -> w133
    tunnel: w132 -> [_ w274 _]
    tunnel: w85 -> [_ w281 _]
    tunnel: w131 -> [_ w275 _]
    tunnel: w130 -> [_ w265 _]
    tunnel: w129 -> [_ w261 _]
    tunnel: w128 -> [_ w255 _]
    tunnel: w127 -> [_ w254 _]
    tunnel: w126 -> [_ w241 _]
    tunnel: w125 -> [_ w240 _]
    tunnel: w124 -> [_ w239 _]
    tunnel: w123 -> [_ w238 _]
    tunnel: w122 -> [_ w237 _]
    tunnel: "Die Number" -> [_ w208 _]
    tunnel: w110 -> [_ w230 _]
    tunnel: w120 -> [_ w223 _]
    tunnel: w87 -> [w197 _ _]
    tunnel: w121 -> [_ w219 _]
    tunnel: w119 -> [_ w207 _]
    tunnel: w68 -> [_ w212 _]
    tunnel: "Light Correction" -> [_ w210 _]
    tunnel: [_ _ w333] -> w117
    tunnel: w116 -> [_ _ w303]
    tunnel: w115 -> [_ _ w305]
    tunnel: w114 -> [_ _ w302]
    tunnel: w113 -> [_ _ w320]
    tunnel: w112 -> [_ _ w321]
    tunnel: w111 -> [_ _ w313]
    tunnel: w83 -> [w195 _ _]
    tunnel: [w169 _ _] -> w82
    tunnel: w79 -> [w177 _ _]
    tunnel: w78 -> [w178 _ _]
    tunnel: w77 -> [w179 _ _]
    tunnel: w76 -> [w180 _ _]
    tunnel: w75 -> [w181 _ _]
    tunnel: w74 -> [w182 _ _]
    tunnel: [w166 _ _] -> w73
    tunnel: w72 -> [w167 _ _]
    tunnel: "Cell Designation" -> [_ w204 _]
    tunnel: w58 -> [_ w200 _]
    frame #0 {
      n38 = Number To Fractional String(number=w177) -> (F-format string=w194:string)  [unwired: 3 out]
      n39 = Number To Fractional String(number=w178) -> (F-format string=w191:string)  [unwired: 3 out]
      n40 = Number To Fractional String(number=w179) -> (F-format string=w190:string)  [unwired: 3 out]
      n41 = Number To Fractional String(number=w180) -> (F-format string=w187:string)  [unwired: 3 out]
      n42 = Number To Fractional String(number=w181) -> (F-format string=w186:string)  [unwired: 3 out]
      n43 = Number To Fractional String(number=w182) -> (F-format string=w183:string)  [unwired: 3 out]
      n44 = Concatenate Strings("Date, " ("concatenated string"), w197) -> (w199:string)
      "Date/Time string" <- w199
      n45 = Concatenate Strings("Session Date, " ("concatenated string"), w167) -> (w166:string)
      n46 = Concatenate Strings("Ambient Temperature (degrees C),  " ("element"), w194) -> (w175:string)
      n47 = Concatenate Strings("Chuck Temperature (degrees C), " ("element"), w191) -> (w174:string)
      n48 = Concatenate Strings("Voc Fit (V), " ("element"), w190) -> (w173:string)
      n49 = Concatenate Strings("Voc Raw (V), " ("element"), w187) -> (w172:string)
      n50 = Concatenate Strings("R at Voc (Ohms), " ("element"), w186) -> (w171:string)
      n51 = Concatenate Strings("R at Isc (Ohms), " ("element"), w183) -> (w176:string)
      n52 = Concatenate Strings("Flash Setup, " ("concatenated string"), w195) -> (w170:string)
      n53 = Build Array(w175, w174, w173, w172, w171, w176, w170) -> (w169:string[])
    }
    frame #1 {
      n54 = Number To Fractional String(number=w277) -> (F-format string=w278:string)  [unwired: 3 out]
      n55 = Number To Fractional String(number=w276) -> (F-format string=w269:string)  [unwired: 3 out]
      n56 = Number To Fractional String(number=w200) -> (F-format string=w201:string)  [unwired: 3 out]
      n57 = Number To Fractional String(number=w299, precision (6)=i16 1) -> (F-format string=w296:string)  [unwired: 2 out]
      n58 = Number To Fractional String(number=w219) -> (F-format string=w221:string)  [unwired: 1 in, 2 out]
      n59 = Number To Fractional String(number=w274) -> (F-format string=w272:string)  [unwired: 3 out]
      n60 = Number To Fractional String(number=w275) -> (F-format string=w291:string)  [unwired: 3 out]
      n61 = Number To Fractional String(number=w265) -> (F-format string=w264:string)  [unwired: 3 out]
      n62 = Number To Fractional String(number=w261) -> (F-format string=w262:string)  [unwired: 3 out]
      n63 = Number To Fractional String(number=w298, precision (6)=i16 1) -> (F-format string=w294:string)  [unwired: 2 out]
      n64 = Number To Fractional String(number=w255) -> (F-format string=w257:string)  [unwired: 3 out]
      n65 = Number To Fractional String(number=w254) -> (F-format string=w259:string)  [unwired: 1 in, 2 out]
      n66 = Number To Fractional String(number=w241, precision (6)=i16 1) -> (F-format string=w242:string)  [unwired: 2 out]
      n67 = Number To Fractional String(number=w240) -> (F-format string=w245:string)  [unwired: 3 out]
      n68 = Number To Fractional String(number=w239) -> (F-format string=w247:string)  [unwired: 3 out]
      n69 = Number To Fractional String(number=w238) -> (F-format string=w250:string)  [unwired: 3 out]
      n70 = Number To Fractional String(number=w237) -> (F-format string=w248:string)  [unwired: 1 in, 2 out]
      n71 = Number To Fractional String(number=w230) -> (F-format string=w231:string)  [unwired: 1 in, 2 out]
      n72 = Concatenate Strings("Device Name, " ("element"), w281) -> (w284:string)
      n73 = Concatenate Strings("Fill Factor, " ("element"), w272) -> (w266:string)
      n74 = Concatenate Strings("Isc (A), " ("string"), w269) -> (w267:string)
      n75 = Concatenate Strings("Voc (V), " ("string"), w278) -> (w268:string)
      n76 = Concatenate Strings("Mask Name, " ("string"), w282) -> (w280:string)
      n77 = Concatenate Strings("Vtest (V), " ("element"), w291) -> (w289:string)
      n78 = Concatenate Strings("Uncorrected Concentration (Suns), " ("element"), w242) -> (w236:string)
      n79 = Concatenate Strings("Comment,  " ("element"), w212) -> (w213:string)
      n80 = Concatenate Strings("Light Correction,  " ("element"), w210) -> (w209:string)
      n81 = Concatenate Strings("X Coord, " ("element"), w296) -> (w288:string)
      n82 = Concatenate Strings("Y Coord, " ("element"), w294) -> (w287:string)
      n83 = Concatenate Strings("Itest (A),  " ("element"), w264) -> (w292:string)
      n84 = Concatenate Strings("Vmax (V),  " ("element"), w262) -> (w260:string)
      n85 = Concatenate Strings("Imax (A),  " ("element"), w257) -> (w253:string)
      n86 = Concatenate Strings("Pmax (W),  " ("element"), w259) -> (w252:string)
      n87 = Concatenate Strings("Corrected Irradiance (W/cm_sq),  " ("element"), w247) -> (w227:string)
      n88 = Concatenate Strings("Equiv 1 sun Jsc,  " ("element"), w221) -> (w217:string)
      n89 = Concatenate Strings("Coating,  " ("element"), w223) -> (w218:string)
      n90 = Concatenate Strings("Package,  " ("element"), w207) -> (w215:string)
      n91 = Concatenate Strings("P_In (W),  " ("element"), w250) -> (w228:string)
      n92 = Concatenate Strings("Efficiency,  " ("element"), w248) -> (w229:string)
      n93 = Concatenate Strings("Isotype Scalar,  " ("element"), w231) -> (w225:string)
      n94 = Concatenate Strings("Hours under test, " ("format string"), w201) -> (w202:string)
      n95 = Concatenate Strings("Cell Designation, " ("element"), w204) -> (w206:string)
      n96 = Concatenate Strings("Die Number, " ("element"), w208) -> (w235:string)
      n97 = Concatenate Strings("Cell Area (cm_sq),  " ("element"), w245) -> (w226:string)
      n98 = Build Array(w280, w284, w206) -> (w286:string[])
      n99 = Build Array (concatenate)(w286, w235, w288, w287, w202, w268, w267, w266, w289, w292, w260, w253, w252, w236, w225, w226, w227, w228, w229, w217, w218, w215, w209, w213) -> (w300:string[])
    }
    frame #2 {
      n100 = Divide(x=w303, y=w305) -> (x/y=w304:dbl)
      n101 = Divide(x=w303, y=w302) -> (x/y=w301:dbl)
      n102 = Number To Fractional String(number=w304) -> (F-format string=w319:string)  [unwired: 3 out]
      n103 = Number To Fractional String(number=w301) -> (F-format string=w325:string)  [unwired: 3 out]
      n104 = Number To Fractional String(number=w303) -> (F-format string=w322:string)  [unwired: 3 out]
      n105 = Number To Fractional String(number=w305) -> (F-format string=w326:string)  [unwired: 3 out]
      n106 = Number To Fractional String(number=w302) -> (F-format string=w328:string)  [unwired: 3 out]
      n107 = Number To Fractional String(number=w320) -> (F-format string=w331:string)  [unwired: 3 out]
      n108 = Number To Fractional String(number=w321) -> (F-format string=w329:string)  [unwired: 1 in, 2 out]
      n109 = Number To Fractional String(number=w313) -> (F-format string=w314:string)  [unwired: 1 in, 2 out]
      n110 = Concatenate Strings("Ratio TopMid, " ("element"), w319) -> (w317:string)
      n111 = Concatenate Strings("Ratio TopBot, " ("element"), w325) -> (w315:string)
      n112 = Concatenate Strings("TopSuns, " ("element"), w322) -> (w311:string)
      n113 = Concatenate Strings("MiddleSuns,  " ("element"), w326) -> (w310:string)
      n114 = Concatenate Strings("Bottom Suns,  " ("element"), w328) -> (w309:string)
      n115 = Concatenate Strings("Error Top,  " ("element"), w331) -> (w308:string)
      n116 = Concatenate Strings("Error Mid,  " ("element"), w329) -> (w307:string)
      n117 = Concatenate Strings("Error Bottom, " ("element"), w314) -> (w306:string)
      n118 = Build Array(w317, w315, w311, w310, w309, w308, w307, w306) -> (w333:string[])
    }
  }
  n119 = Open/Create/Replace File(file path (use dialog)=w88, error in="error in", operation (0:open)=T9."open or create") -> (refnum out=w38:refnum<file>, error out=w37:errorcluster)  [unwired: 2 in, 2 out]
  n120 = Index Array(array="IV array", index (row) #1=0 ("index (row)"), index (row) #2=1 ("index (row)"), index (row) #3=2 ("index (row)"), index (row) #4=3 ("index (row)")) -> (element #1=w27:dbl[], element #2=w25:dbl[], element #3=w24:dbl[], element #4=w1:dbl[])  [unwired: 4 in]
  n121 = case shown="True" TRUE {
    tunnel: w37 -> [w334 w340]
    tunnel: [w334 w339] -> w36
    tunnel: w38 -> [w335 w337]
    tunnel: [w335 w338] -> w35
    frame False {
    }
    frame True {
      n122 = Set File Position(refnum=w337, from (0:start)=enum16{"start", "end", "current"}."end", error in=w340) -> (refnum out=w338:refnum<file>, error out=w339:errorcluster)  [unwired: 1 out]
    }
  }
  n123 = Array To Spreadsheet String(delimiter (Tab)=w2, array=w27, 3:"%.5e") -> (spreadsheet string=w22:string)
  n124 = Concatenate Strings("V, " ("string"), w22) -> (w16:string)
  n125 = Build Array (concatenate)(w73, w133, w134, w82, w117) -> (w137:string[])
  n126 = Write to Text File(file (use dialog)=w35, text=w137, error in=w36) -> (refnum out=w33:refnum<file>, error out=w32:errorcluster)  [unwired: 1 in, 1 out]
  n127 = Array To Spreadsheet String(delimiter (Tab)=w2, array=w25, 3:"%.5e") -> (spreadsheet string=w21:string)
  n128 = Write to Text File(file (use dialog)=w33, text=w16, error in=w32) -> (refnum out=w13:refnum<file>, error out=w11:errorcluster)  [unwired: 2 out]
  n129 = Concatenate Strings("I, " ("string"), w21) -> (w15:string)
  n130 = Write to Text File(file (use dialog)=w13, text=w15, error in=w11) -> (refnum out=w12:refnum<file>, error out=w10:errorcluster)  [unwired: 2 out]
  n131 = Array To Spreadsheet String(delimiter (Tab)=w2, array=w24, 3:"%.5e") -> (spreadsheet string=w20:string)
  n132 = Concatenate Strings("P, " ("string"), w20) -> (w14:string)
  n133 = Write to Text File(file (use dialog)=w12, text=w14, error in=w10) -> (refnum out=w7:refnum<file>, error out=w6:errorcluster)  [unwired: 2 out]
  n134 = Array To Spreadsheet String(delimiter (Tab)=w2, array=w1, 3:"%.5e") -> (spreadsheet string=w3:string)
  n135 = Concatenate Strings("Iraw, " ("string"), w3) -> (w8:string)
  n136 = Write to Text File(file (use dialog)=w7, text=w8, error in=w6) -> (refnum out=w4:refnum<file>, error out=w5:errorcluster)  [unwired: 2 out]
  n137 = Close File(refnum=w4, error in=w5) -> (error out=→"error out":errorcluster)  [unwired: 1 out]
